vi "LVRT test.vi"() -> ()   [LabVIEW 2017]
uses:
  <vilib>/FPGAPlugInAG/cRIO-9068/niLvFpga_Open_cRIO-9068.vi
  <vilib>/rvi/interface/common/dynamic/niFpgaDynamicAddResources.vi
  <vilib>/Utility/error.llb/Error Cluster From Error Code.vi
  <vilib>/rvi/errors/niLvFpgaAdjustHostInterfaceError.vi
  <vilib>/RVI Host/nirviSupport.llb/nirviErrorClusterFromErrorCode.vi
  <vilib>/FPGAPlugInAG/Dynamic/niLvFpga_Close_Dynamic.vi
  <vilib>/rvi/interface/nirviOpenFPGA/nirviOpenFPGA.xnode
  FPGA Bitfiles/FPGACommunicatio_FPGATarget_FPGA_k2pYpE7HhZg.lvbitx
  FPGA.vi
  <vilib>/rvi/interface/nirviMethod/nirviMethod.xnode
  <vilib>/rvi/interface/nirviReadWriteControl/nirviReadWriteControl.xnode
  <vilib>/rvi/interface/nirviCloseFPGA/nirviCloseFPGA.xnode
  NiFpgaLv.dll
  <vilib>/rvi/interface/Simulation/niFpgaSimulationCallBeginRW.vi
  <vilib>/FPGAPlugInAG/Dynamic/niLvFpga_ReadFifo_Dynamic.vi
  <vilib>/rvi/errors/niLvFpgaMergeErrorWithErrorCode.vi
  <vilib>/rvi/interface/nirviMethod/StockFPGA_InlinedMethodWaitForSingleIRQ.vi
  <vilib>/FPGAPlugInAG/Dynamic/niLvFpga_WaitOnIrq_Dynamic.vi
  <vilib>/FPGAPlugInAG/Dynamic/niLvFpga_AcknowledgeIrq_Dynamic.vi
panel:
  out "Elements Remaining":u32
  in  "Read Noise?":bool
  in  "FIFO elements to read":u32
  in  "stop":bool
  out "Data":i16[](array[numeric])
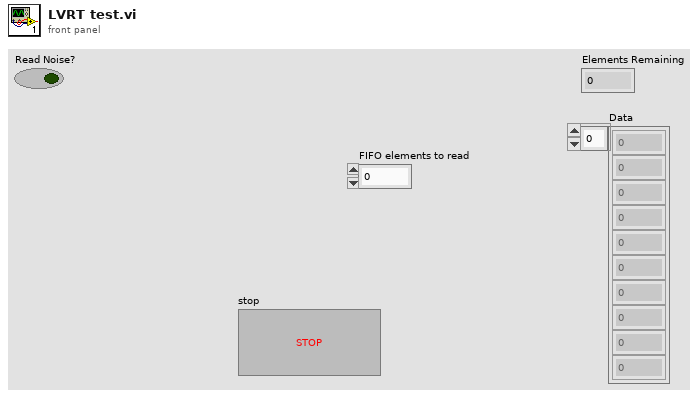
[diagram p1: front panel]
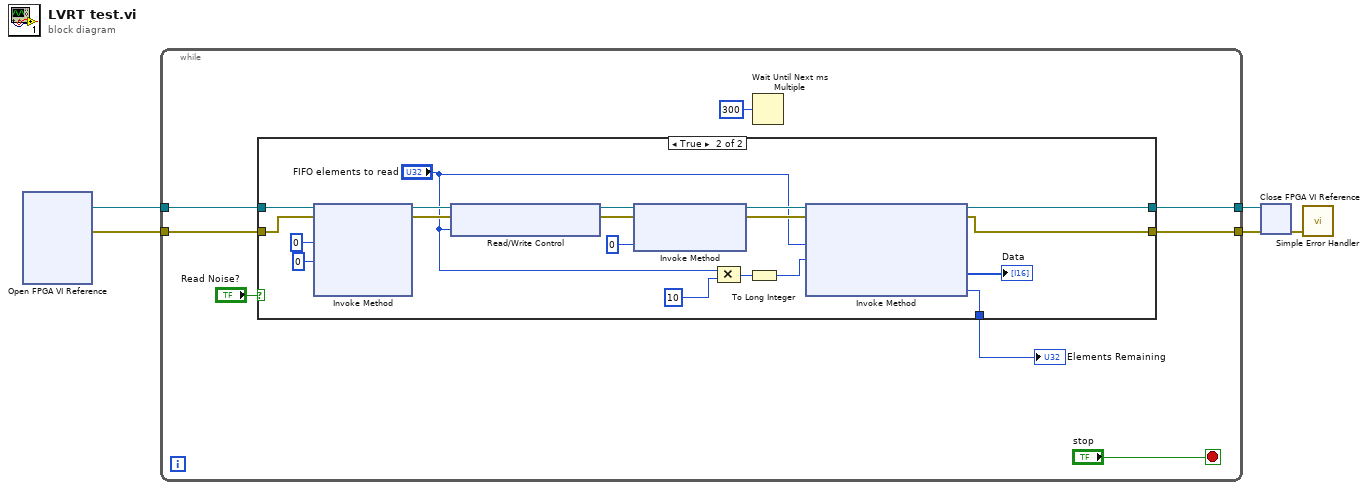
[diagram p0: block diagram]
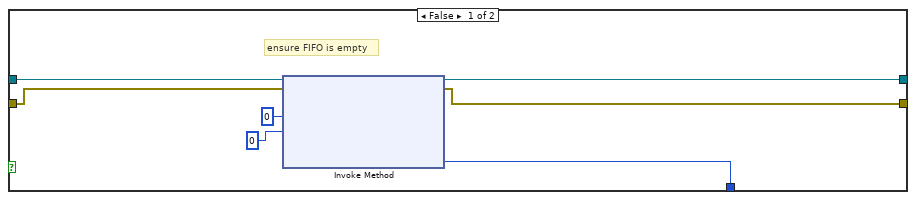
[diagram p2: hidden frame]
diagram:
  n1 = xnode "Open FPGA VI Reference"() -> ("FPGA VI Reference Out"=w5:refnum<k20>, "error out"=w4:errorcluster)  [unwired: 2 in]
  n2 = while {
    tunnel: w5 -> [w11]
    tunnel: w4 -> [w9]
    tunnel: [w8] -> w2
    tunnel: [w7] -> w1
    stop <- "stop" stop-if-true
    n3 = case shown="True" "Read Noise?" {
      tunnel: w11 -> [w20 w39]
      tunnel: w9 -> [w19 w35]
      tunnel: [w15 w23] -> w8
      tunnel: [w16 w22] -> w7
      tunnel: [w14 w21] -> w6
      frame False {
        # "ensure FIFO is empty"
        n4 = xnode "Invoke Method"("FPGA VI Reference In"=w20, "error in"=w19, "Number of Elements"=u32 0, "Timeout (ms)"=0) -> ("FPGA VI Reference Out"=w15:refnum<k20>, "error out"=w16:errorcluster, "Elements Remaining"=w14:u32)  [unwired: 1 out]
      }
      frame True {
        n5 = xnode "Invoke Method"("FPGA VI Reference In"=w39, "error in"=w35, "IRQ Number(s)"=0, "Timeout (ms)"=0) -> ("FPGA VI Reference Out"=w34:refnum<k20>, "error out"=w33:errorcluster)  [unwired: 2 out]
        n6 = xnode "Read/Write Control"("FPGA VI Reference In"=w34, "error in"=w33, "White Noise Data Length"="FIFO elements to read") -> ("FPGA VI Reference Out"=w32:refnum<k20>, "error out"=w31:errorcluster)
        n7 = xnode "Invoke Method"("FPGA VI Reference In"=w32, "error in"=w31, "IRQ Number(s)"=0) -> ("FPGA VI Reference Out"=w30:refnum<k20>, "error out"=w29:errorcluster)
        n8 = Compound Arithmetic op=MULTIPLY("FIFO elements to read", u32 10 ("value")) -> (w26:u32)
        n9 = To Long Integer(number=w26) -> (32bit integer=w25:i32)
        n10 = xnode "Invoke Method"("FPGA VI Reference In"=w30, "error in"=w29, "Number of Elements"="FIFO elements to read", "Timeout (ms)"=w25) -> ("FPGA VI Reference Out"=w23:refnum<k20>, "error out"=w22:errorcluster, "Data"=→"Data":i16[], "Elements Remaining"=w21:u32)
      }
    }
    "Elements Remaining" <- w6
    n11 = Wait Until Next ms Multiple(millisecond multiple=u32 300) -> ()  [unwired: 1 out]
  }
  n12 = xnode "Close FPGA VI Reference"("FPGA VI Reference In"=w2, "error in"=w1) -> ("error out"=w3:errorcluster)
  n13 = call <vilib>:"Simple Error Handler.vi"("error in (no error)"=w3) -> ()  [unwired: 4 in, 5 out]
